vi "Match Name.vi"(6 "Exact (T)":bool=TRUE, 8 "error in (no error)":errorcluster, 10 "Name":string, 11 "Config Lookup (New)":refnum<class "Config Lookup.lvclass">) -> (0 "error out":errorcluster, 3 "Config Lookup out":refnum<class "Config Lookup.lvclass">)   [LabVIEW 2020, in "CDM-Config.lvlib" / "Config Lookup.lvclass"]
doc: "Specifies the name an element must be set to in order to match in a lookup. An element's name is always the last element in its hierarchy array. When doing descendent lookup, multiple elements can be matched. When doing an ancestor lookup, the first element that matches the name will be returned."
uses:
  Config Filter/Config Lookup.lvclass
  Config Filter/Config Lookup.lvclass/Config Lookup.ctl
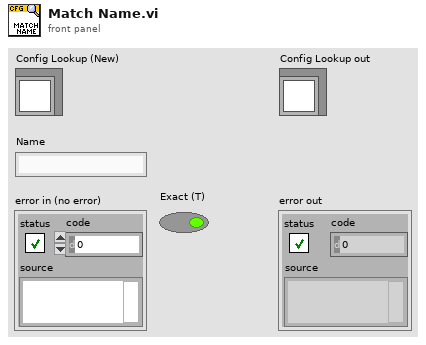
[diagram p1: front panel]
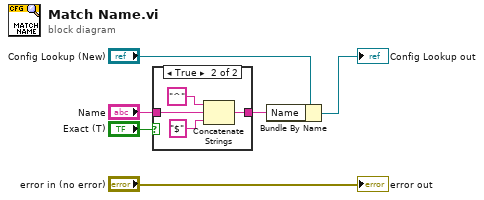
[diagram p0: block diagram]
diagram:
  n1 = case shown="True" "Exact (T)" {
    tunnel: "Name" -> [w7 w11]
    tunnel: [w7 w10] -> w2
    frame False {
    }
    frame True {
      n2 = Concatenate Strings("^" ("string"), w11, "$" ("string")) -> (w10:string)
    }
  }
  n3 = Bundle By Name(cluster="Config Lookup (New)", "Name"=w2) -> (→"Config Lookup out":refnum<class "Config Lookup.lvclass">)
  "error out" <- "error in (no error)"
